vi "Stimulus-Enumerate Valid Params.vi"(0 "Stimulus Channel (Full)":T22(xcontrol), 11 "error in (no error)":errorcluster) -> (4 "Parameter Names":string[](array[string]), 15 "error out":errorcluster)   [LabVIEW 2015]
uses:
  Controls/Waveform XCtl/Waveform Enum.ctl
  Controls/Stimulus Channel (Full)/Stimulus Channel (Full).xctl
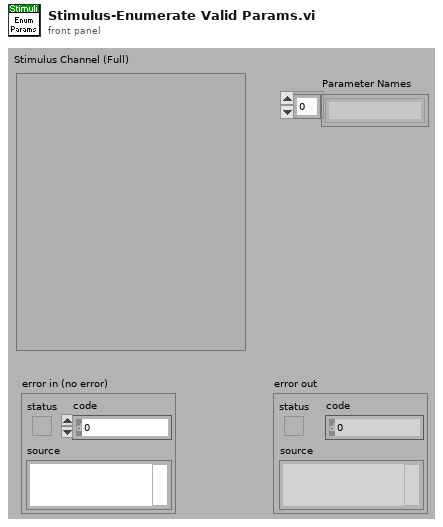
[diagram p1: front panel]
types:
  T1 = typedef "Waveform XCtl.xctl/Waveform Data.ctl" = cluster{"Type":T2, "Tone":T3, "Pulse Train":T4, "Noise":T7, "File":T8, "FMSweep":T9, "Chirp Train":T10, "Complex Tone":cluster{"Params":T12, "Data":T14}}
  T2 = typedef "Waveform Enum.ctl" = enum16{"OFF", "Tone", "Noise", "Pulse Train", "File", "FM Sweep", "Chirp Train", "Complex Tone", "FM Tone"}
  T3 = typedef "Tone Params.ctl" = cluster{"Frequency (kHz)":dbl, "Last Freq":dbl, "Last Phase":dbl}
  T4 = typedef "Pulse Train Params.ctl" = cluster{"Pulse width (us)":dbl, "Pulse rate (Hz)":dbl, "Gap (ms)":dbl, "Polarity":T5, "PT State":T6, "Asynch":bool}
  T5 = typedef "Pulse Polarity.ctl" = enum16{"POS", "NEG", "POS-NEG", "NEG-POS"}
  T6 = typedef "PT-Continuous State.ctl" = cluster{"Template":dbl[], "Nperiod":i32, "Index":i32, "Pulse Rate (Hz)":dbl, "Phase (cycles)":dbl, "Noff":i32}
  T7 = typedef "Noise Params.ctl" = cluster{"InvFilt":bool, "Noise":dbl[], "CurPt":i32, "Aweight":bool, "Seed":i32, "afile":path}
  T8 = typedef "StimFile-Params.ctl" = cluster{"Filename":path, "Signal":dbl[], "Channel":i32}
  T9 = typedef "FM Sweep Params.ctl" = cluster{"Rate (oct/s)":dbl, "Fmin (Hz)":dbl, "Fmax (Hz)":dbl, "Ramp (ms)":dbl, "Linear":bool}
  T10 = typedef "Chirp Train.ctl" = cluster{"Params":T11, "Data":cluster{"WF":dbl[]}}
  T11 = typedef "Chirp Train Params.ctl" = cluster{"Fmin (kHz)":dbl, "Fmax (kHz)":dbl, "Compensate":bool, "Duration (ms)":dbl}
  T12 = typedef "CT-Params.ctl" = cluster{"F0 (Hz)":dbl, "Band":cluster{"Flow (Hz)":dbl, "Fhigh (Hz)":dbl}, "Phase":T13, "Min F0 (Hz)":dbl, "Max F0 (Hz)":dbl, "ContinRandPhase":bool, "Max peak factor":dbl, "Max mod depth":dbl, "MinHarmNum":i32, "MaxHarmNum":i32, "Level Mode":enum16{"per component", "overall rms"}, "% jitter":dbl}
  T13 = typedef "CT-Phase Enum.ctl" = enum16{"Cosine", "Random", "Alternating"}
  T14 = typedef "CT-Runtime Data.ctl" = cluster{"Ncomp":i32, "MinHarm":i32, "Phase":dbl[], "Amplitude":dbl[], "Npts/frame":i32, "Last F0":dbl, "Fmin":dbl, "Fmax":dbl, "Lslope":dbl, "randphase":bool, "overall rms":bool, "fmult":dbl[], "jittered":bool}
  T15 = typedef "Advanced Filter XCtl.xctl/Filter Data.ctl" = cluster{"Type":enum16{"Lowpass", "Highpass", "Bandpass", "Bandstop", "OFF"}, "CF (kHz)":dbl, "BW (kHz)":dbl, "Cascade":bool, "Quadrature":bool, "Scale Factor":dbl, "Stages":cluster{"IIR Filter":cluster{"filter structure":enum32{"IIR 2nd Order", "IIR 4th Order"}, "Reverse Coefficients":dbl[], "Forward Coefficients":dbl[]}, "State":dbl[]}[], "Class":enum16{"Elliptic", "Butterworth"}, "Order":i32, "BWUnits":T16}
  T16 = typedef "Filter-Bandwidth Units.ctl" = enum16{"Linear", "Octaves", "Min-Max"}
  T17 = typedef "Burst Control.xctl/Burst Data.ctl" = cluster{"Active":bool, "Delay (ms)":dbl, "Duration (ms)":dbl, "Ramp (ms)":dbl, "Rate (Hz)":dbl, "Trepeat (ms)":dbl, "Repeat":bool}
  T18 = typedef "Level XCtl.xctl/Level Data.ctl" = cluster{"Level":dbl, "Units":T19, "Max":dbl, "Multiplier":dbl, "Cal File":path, "Cal":cluster{"Freq (Hz)":dbl[], "Mag (dB SPL)":dbl[], "Phase (deg)":dbl[]}}
  T19 = typedef "Level Units.ctl" = enum16{"dB atten", "dB SPL", "dB re 1 Vrms", "dB V/Hz½", "mW", "dB SL"}
  T20 = typedef "Advanced Stimulus Options.xctl/Advanced Stimulus Options.ctl" = cluster{"Rep Mask":string, "AltPol":bool, "Var":string, "Expr":string}
  T21 = typedef "SAM Params.ctl" = cluster{"Active":bool, "Frequency (Hz)":dbl, "Depth":dbl, "Init Phase (cycles)":dbl, "phase (degrees)":dbl, "Asynch":bool}
  T22 = cluster{"Waveform":T1, "Filter":T15, "Burst":T17, "Level":T18, "Name":string, "Advanced":T20, "SAM":T21}
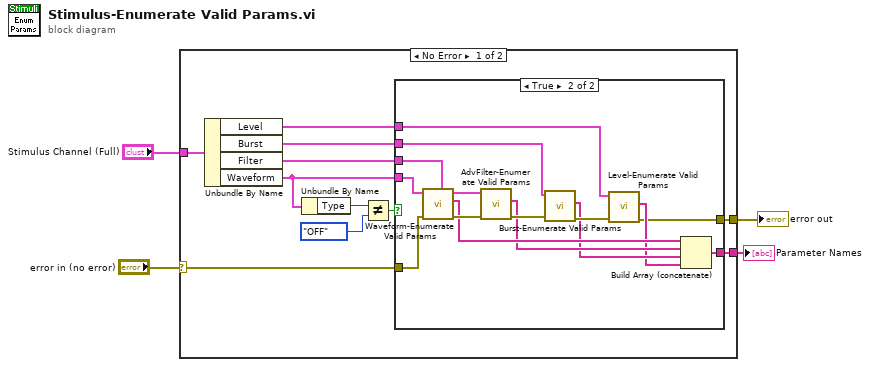
[diagram p0: block diagram]
diagram:
  n1 = case shown="No Error" "error in (no error)" {
    selector: "error in (no error)" -> [w7 w31]
    tunnel: "Stimulus Channel (Full)" -> [w15 _]
    tunnel: [w8 _] -> w3
    tunnel: [w6 w31] -> w1
    frame No Error {
      n2 = Unbundle By Name(w15) -> ("Level"=w12:T18, "Burst"=w13:T17, "Filter"=w14:T15, "Waveform"=w11:T1)
      n3 = Unbundle By Name(w11) -> ("Type"=w10:T2)
      n4 = Not Equal?(x=w10, y=Waveform_Enum."OFF") -> (x != y?=w5:bool)
      n5 = case shown="True" w5 {
        tunnel: w14 -> [_ w28]
        tunnel: w13 -> [_ w27]
        tunnel: w12 -> [_ w25]
        tunnel: w11 -> [_ w24]
        tunnel: [_ w19] -> w8
        tunnel: w7 -> [w16 w18]
        tunnel: [w16 w17] -> w6
        frame False {
        }
        frame True {
          n6 = call "Waveform-Enumerate Valid Params.vi"("error in (no error)"=w18, "Waveform"=w24) -> ("error out"=w30:errorcluster, "Parameter Names"=w23:string[])  [unwired: 8 in]
          n7 = call "AdvFilter-Enumerate Valid Params.vi"("error in (no error)"=w30, "Filter"=w28) -> ("error out"=w29:errorcluster, "Parameter Names"=w22:string[])  [unwired: 8 in]
          n8 = call "Burst-Enumerate Valid Params.vi"("error in (no error)"=w29, "Burst"=w27) -> ("error out"=w26:errorcluster, "Parameter Names"=w21:string[])  [unwired: 8 in]
          n9 = call "Level-Enumerate Valid Params.vi"("error in (no error)"=w26, "Level"=w25) -> ("error out"=w17:errorcluster, "Parameter Names"=w20:string[])  [unwired: 8 in]
          n10 = Build Array (concatenate)(w23, w22, w21, w20) -> (w19:string[])
        }
      }
    }
    frame Error {
    }
  }
  "error out" <- w1
  "Parameter Names" <- w3
